vi "Hardware - ECS - EPTx Host.vi"() -> ()   [LabVIEW 2015, in "ECS-Host.lvlib"]
uses:
  ECS-Host.lvlib
  Typedefs/EPT/Engine Status.ctl
  Typedefs/EPT/Digital Channel Assignment - ECS.ctl
  ECS-Shared.lvlib
panel:
  in  "SimKnockResult":u8
  in  "PrimaryIndex":u8
  in  "Aux1Index":u8
  in  "Aux2Index":u8
  in  "Aux3Index":u8
  in  "Aux4Index":u8
  in  "PrimaryIndex2":u8
  in  "Aux1Index2":u8
  in  "Aux2Index2":u8
  in  "Aux3Index2":u8
  in  "Aux4Index2":u8
  out "EngineStatus":u8
  out "KnockResult":u8
  in  "GateReset":u8
  in  "EncoderB":u8
  in  "EncoderZ":u8
  in  "EncoderA":u8
  in  "_EPT Tab Control":T1(tab)
  in  "ForceSafeState":bool
  in  "MaxSampleRate":sgl caption="[Hz]" format="%#.3p"
  in  "EncToothCount":u32 caption="[ppr]"
  out "CurrentCAD":sgl caption="CAD" max=200 step=1
  out "ConfigFPGA2":bool caption="FPGA2Write"
  out "ConfigFPGA1":bool caption="FPGA1Write"
  in  "Aux4Filt":sgl caption="[s]" format="%#.3f"
  in  "Aux3Filt":sgl caption="[s]" format="%#.3f"
  in  "Aux2Filt":sgl caption="[s]" format="%#.3f"
  in  "Aux1Filt":sgl caption="[s]" format="%#.3f"
  in  "PrimaryFilt":sgl caption="[s]" format="%#.3f"
  out "ReceivingPrimaryFPGA2":bool caption="RCVG PRIMARY"
  out "ReceivingPrimaryFPGA1":bool caption="RCVG PRIMARY"
  out "StalledFPGA2":bool
  out "StalledFPGA1":bool
  out "AuxWarningFPGA2":bool
  out "EPTxErrorFPGA2":bool
  out "AuxWarningFPGA1":bool
  in  "SimEnable":bool
  in  "_GateReset":T2 caption="GateReset" items=["Not Selected", "9411 Chan 0", "9411 Chan 1", "9411 Chan 2", "9411 Chan 3", "9411 Chan 4", "9411 Chan 5", "AD Combo VR 1", "AD Combo VR 2", "AD Combo Hall 1", "AD Combo Hall 2"]
  in  "_EncoderZ":T2 caption="EncoderZ" items=["Not Selected", "9411 Chan 0", "9411 Chan 1", "9411 Chan 2", "9411 Chan 3", "9411 Chan 4", "9411 Chan 5", "AD Combo VR 1", "AD Combo VR 2", "AD Combo Hall 1", "AD Combo Hall 2"]
  in  "_EncoderB":T2 caption="EncoderB" items=["Not Selected", "9411 Chan 0", "9411 Chan 1", "9411 Chan 2", "9411 Chan 3", "9411 Chan 4", "9411 Chan 5", "AD Combo VR 1", "AD Combo VR 2", "AD Combo Hall 1", "AD Combo Hall 2"]
  out "SyncFPGA2":bool caption="FPGA2Sync"
  out "FPGA1Error":bool caption="FPGA1Interface"
  out "FPGA2Error":bool caption="FPGA2Interface"
  out "EngineSpeedFPGA2":sgl caption="RPM" min=0 max=0.2 step=0.001 format="%#.3f"
  in  "EncSignalSelect":bool caption="CASEncSignalSelect"
  out "WatchdogErrorFPGA1":bool
  out "OverflowFPGA1":bool
  out "PatternErrorFPGA1":bool
  out "RatioErrorFPGA1":bool
  in  "CrankRunThreshold":sgl caption="RPM" format="%#.3f"
  in  "StallSpeed":sgl caption="RPM" format="%#.3f"
  out "SyncFPGA1":bool caption="FPGA1Sync"
  out "EngineSpeedFPGA1":sgl caption="RPM" min=0 max=0.2 step=0.001 format="%#.3f"
  out "MaxCAD":sgl caption="CAD" max=200 step=1
  out "_Engine Status":T3 caption="Engine Status"
  in  "SimulatedSpeed":sgl caption="RPM" format="%#.3f"
  in  "ClearEPTxErrors":bool
  in  "SyncEnable":bool
  in  "_EncoderA":T2 caption="EncoderA" items=["Not Selected", "9411 Chan 0", "9411 Chan 1", "9411 Chan 2", "9411 Chan 3", "9411 Chan 4", "9411 Chan 5", "AD Combo VR 1", "AD Combo VR 2", "AD Combo Hall 1", "AD Combo Hall 2"]
  in  "SettingsFilename":string
  in  "ReloadEPTxSettings":bool
  out "LoadingFPGA1":bool caption="Status"
  in  "_Dig Select Tabs":enum32{"FPGA1", "FPGA2"}(tab)
  in  "_Aux4Index":T2 caption="Aux4Index" items=["Not Selected", "9411 Chan 0", "9411 Chan 1", "9411 Chan 2", "9411 Chan 3", "9411 Chan 4", "9411 Chan 5", "AD Combo VR 1", "AD Combo VR 2", "AD Combo Hall 1", "AD Combo Hall 2"]
  in  "_Aux3Index":T2 caption="Aux3Index" items=["Not Selected", "9411 Chan 0", "9411 Chan 1", "9411 Chan 2", "9411 Chan 3", "9411 Chan 4", "9411 Chan 5", "AD Combo VR 1", "AD Combo VR 2", "AD Combo Hall 1", "AD Combo Hall 2"]
  in  "_Aux2Index":T2 caption="Aux2Index" items=["Not Selected", "9411 Chan 0", "9411 Chan 1", "9411 Chan 2", "9411 Chan 3", "9411 Chan 4", "9411 Chan 5", "AD Combo VR 1", "AD Combo VR 2", "AD Combo Hall 1", "AD Combo Hall 2"]
  in  "_Aux1Index":T2 caption="Aux1Index" items=["Not Selected", "9411 Chan 0", "9411 Chan 1", "9411 Chan 2", "9411 Chan 3", "9411 Chan 4", "9411 Chan 5", "AD Combo VR 1", "AD Combo VR 2", "AD Combo Hall 1", "AD Combo Hall 2"]
  in  "_PrimaryIndex":T2 caption="PrimaryIndex" items=["Not Selected", "9411 Chan 0", "9411 Chan 1", "9411 Chan 2", "9411 Chan 3", "9411 Chan 4", "9411 Chan 5", "AD Combo VR 1", "AD Combo VR 2", "AD Combo Hall 1", "AD Combo Hall 2"]
  in  "_Aux4Index2":T2 caption="Aux4Index" items=["Not Selected", "9411 Chan 0", "9411 Chan 1", "9411 Chan 2", "9411 Chan 3", "9411 Chan 4", "9411 Chan 5", "AD Combo VR 1", "AD Combo VR 2", "AD Combo Hall 1", "AD Combo Hall 2"]
  in  "_Aux3Index2":T2 caption="Aux3Index" items=["Not Selected", "9411 Chan 0", "9411 Chan 1", "9411 Chan 2", "9411 Chan 3", "9411 Chan 4", "9411 Chan 5", "AD Combo VR 1", "AD Combo VR 2", "AD Combo Hall 1", "AD Combo Hall 2"]
  in  "_Aux2Index2":T2 caption="Aux2Index" items=["Not Selected", "9411 Chan 0", "9411 Chan 1", "9411 Chan 2", "9411 Chan 3", "9411 Chan 4", "9411 Chan 5", "AD Combo VR 1", "AD Combo VR 2", "AD Combo Hall 1", "AD Combo Hall 2"]
  in  "_Aux1Index2":T2 caption="Aux1Index" items=["Not Selected", "9411 Chan 0", "9411 Chan 1", "9411 Chan 2", "9411 Chan 3", "9411 Chan 4", "9411 Chan 5", "AD Combo VR 1", "AD Combo VR 2", "AD Combo Hall 1", "AD Combo Hall 2"]
  in  "_PrimaryIndex2":T2 caption="PrimaryIndex" items=["Not Selected", "9411 Chan 0", "9411 Chan 1", "9411 Chan 2", "9411 Chan 3", "9411 Chan 4", "9411 Chan 5", "AD Combo VR 1", "AD Combo VR 2", "AD Combo Hall 1", "AD Combo Hall 2"]
  in  "AuxTTL-3TDC":T4(ring)
  in  "AuxTTL-4TDC":T4(ring)
  in  "AuxTTL-7TDC":T4(ring)
  in  "AuxTTL-8TDC":T4(ring)
  in  "AuxTTL-2TDC":T4(ring)
  in  "AuxTTL-1TDC":T4(ring)
  in  "AuxTTL-5TDC":T4(ring)
  in  "AuxTTL-6TDC":T4(ring)
  in  "Spark1-3TDC":T4(ring)
  in  "Spark1-4TDC":T4(ring)
  in  "Spark1-7TDC":T4(ring)
  in  "Spark1-8TDC":T4(ring)
  in  "Spark1-2TDC":T4(ring)
  in  "Spark1-1TDC":T4(ring)
  in  "Spark1-5TDC":T4(ring)
  in  "Spark1-6TDC":T4(ring)
  in  "DI1-2TDC":T4(ring)
  in  "DI1-1TDC":T4(ring)
  in  "DI2-2TDC":T4(ring)
  in  "DI2-1TDC":T4(ring)
  in  "DI4-2TDC":T4(ring)
  in  "DI4-1TDC":T4(ring)
  in  "DI3-2TDC":T4(ring)
  in  "DI3-1TDC":T4(ring)
  in  "GlobalTDCOffset":sgl caption="CAD" min=0 max=0.2 step=0.001 format="%#.3f"
  in  "TDC1":sgl caption="CAD" min=0 max=720 step=0.001 format="%#.3f"
  in  "TDC2":sgl caption="CAD" min=0 max=720 step=0.001 format="%#.3f"
  in  "TDC3":sgl caption="CAD" min=0 max=720 step=0.001 format="%#.3f"
  in  "TDC4":sgl caption="CAD" min=0 max=0.2 step=0.001 format="%#.3f"
  in  "TDC5":sgl caption="CAD" min=0 max=0.2 step=0.001 format="%#.3f"
  in  "TDC6":sgl caption="CAD" min=0 max=0.2 step=0.001 format="%#.3f"
  in  "TDC7":sgl caption="CAD" min=0 max=0.2 step=0.001 format="%#.3f"
  in  "TDC8":sgl caption="CAD" min=0 max=0.2 step=0.001 format="%#.3f"
  in  "PFI1-3TDC":T4(ring)
  in  "PFI1-4TDC":T4(ring)
  in  "PFI2-3TDC":T4(ring)
  in  "PFI2-4TDC":T4(ring)
  in  "PFI1-2TDC":T4(ring)
  in  "PFI1-1TDC":T4(ring)
  in  "PFI2-1TDC":T4(ring)
  in  "PFI2-2TDC":T4(ring)
  out "Aux4EdgeCount":sgl caption="[DBTDC]"
  out "Aux3EdgeCount":sgl caption="[]"
  out "Aux2EdgeCount":sgl caption="[]"
  out "Aux1EdgeCount":sgl caption="[]"
  out "Aux4Adv":sgl caption="[CAD]" format="%#.2f"
  in  "Aux4DefaultPsn":sgl caption="[DBTDC]" format="%#.2f"
  out "Aux4RisingEdge":sgl caption="[DBTDC]"
  in  "Aux4CaptureStart":sgl caption="[DBTDC]" format="%#.2f"
  in  "Aux4CaptureEnd":sgl caption="[DBTDC]" format="%#.2f"
  out "Aux3Adv":sgl caption="[CAD]" format="%#.2f"
  in  "Aux3DefaultPsn":sgl caption="[DBTDC]" format="%#.2f"
  out "Aux3RisingEdge":sgl caption="[]"
  in  "Aux3CaptureStart":sgl caption="[DBTDC]" format="%#.2f"
  in  "Aux3CaptureEnd":sgl caption="[]" format="%#.2f"
  out "Aux2Adv":sgl caption="[CAD]" format="%#.2f"
  out "Aux1Adv":sgl caption="[CAD]" format="%#.2f"
  in  "Aux2DefaultPsn":sgl caption="[DBTDC]" format="%#.2f"
  in  "Aux1DefaultPsn":sgl caption="[DBTDC]" format="%#.2f"
  out "Aux2RisingEdge":sgl caption="[]"
  out "Aux1RisingEdge":sgl caption="[]"
  in  "Aux1CaptureStart":sgl caption="[DBTDC]" format="%#.2f"
  in  "Aux1CaptureEnd":sgl caption="[]" format="%#.2f"
  in  "Aux2CaptureStart":sgl caption="[DBTDC]" format="%#.2f"
  in  "Aux2CaptureEnd":sgl caption="[]" format="%#.2f"
  in  "VVT-TDCRef":T5(ring)
  in  "SimKnockEnable":bool
  in  "_SimKnockResult":bool[](array[boolean]) caption="SimKnockResult"
  in  "Knock-6TDC":T4(ring)
  in  "Knock-8TDC":T4(ring)
  in  "Knock-4TDC":T4(ring)
  in  "Knock-2TDC":T4(ring)
  in  "Knock-1TDC":T4(ring)
  in  "Knock-5TDC":T4(ring)
  in  "Knock-3TDC":T4(ring)
  in  "Knock-7TDC":T4(ring)
  in  "KnockSensorCyl3":T4(ring)
  in  "KnockSensorCyl4":T4(ring)
  in  "KnockSensorCyl7":T4(ring)
  in  "KnockSensorCyl8":T4(ring)
  in  "KnockSensorCyl2":T4(ring)
  in  "KnockSensorCyl1":T4(ring)
  in  "KnockSensorCyl5":T4(ring)
  in  "KnockSensorCyl6":T4(ring)
  in  "KnockRefWindowEnd":sgl caption="[DBTDC]"
  in  "KnockRefWindowStart":sgl caption="[DBTDC]"
  in  "KnockWindowEnd":sgl caption="[DBTDC]"
  in  "KnockWindowStart":sgl caption="[DBTDC]"
  in  "KnockThreshold":sgl caption="[]"
  in  "KnockHighCutoff":sgl caption="[Hz]"
  in  "KnockLowCutoff":sgl caption="[Hz]"
  in  "KnockFrequency":sgl caption="[Hz]"
  out "KnockIntensity":sgl[](array[numeric])
  out "_Knock":bool[](array[boolean]) caption="Knock"
  # "FPGA1"
  # "FPGA2"
  # "FPGA1"
  # "FPGA2"
  # "Sim Encoder\nResolution"
  # "Max CAS DAQ\nSample Rate"
  # "Digital Signal and Filter Select"
  # "AUX 1"
  # "AUX 2"
  # "AUX 3"
  # "AUX 4"
  # "CaptureStart"
  # "CaptureEnd"
  # "RisingEdge"
  # "EdgeCount"
  # "DefaultPosition"
  # "Advance"
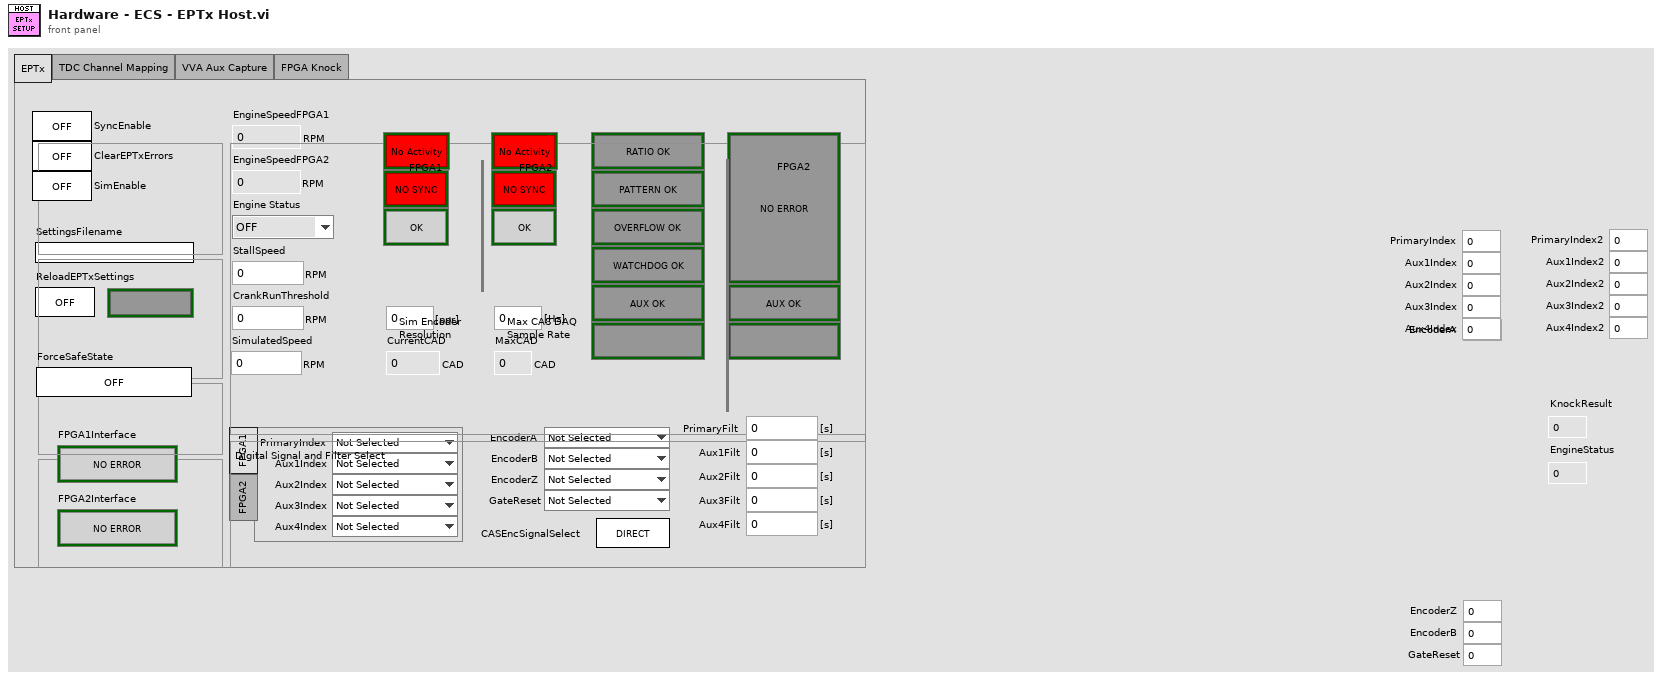
[diagram p1: front panel]
types:
  T1 = enum32{"EPTx", "TDC Channel Mapping", "VVA Aux Capture", "FPGA Knock"}
  T2 = typedef "ECS-Shared.lvlib/Digital Channel Assignment - ECS.ctl" = u8
  T3 = typedef "ECS-Shared.lvlib/Engine Status.ctl" = enum16{"OFF", "STALLED", "CRANKING", "RUNNING", "ACCEL", "DECEL", "SAFE"}
  T4 = enum32{"TDC1", "TDC2", "TDC3", "TDC4", "TDC5", "TDC6", "TDC7", "TDC8", "TDC9", "TDC10", "TDC11", "TDC12"}
  T5 = enum32{"TDC1", "TDC2", "TDC3", "TDC4", "TDC5", "TDC6", "TDC7", "TDC8"}
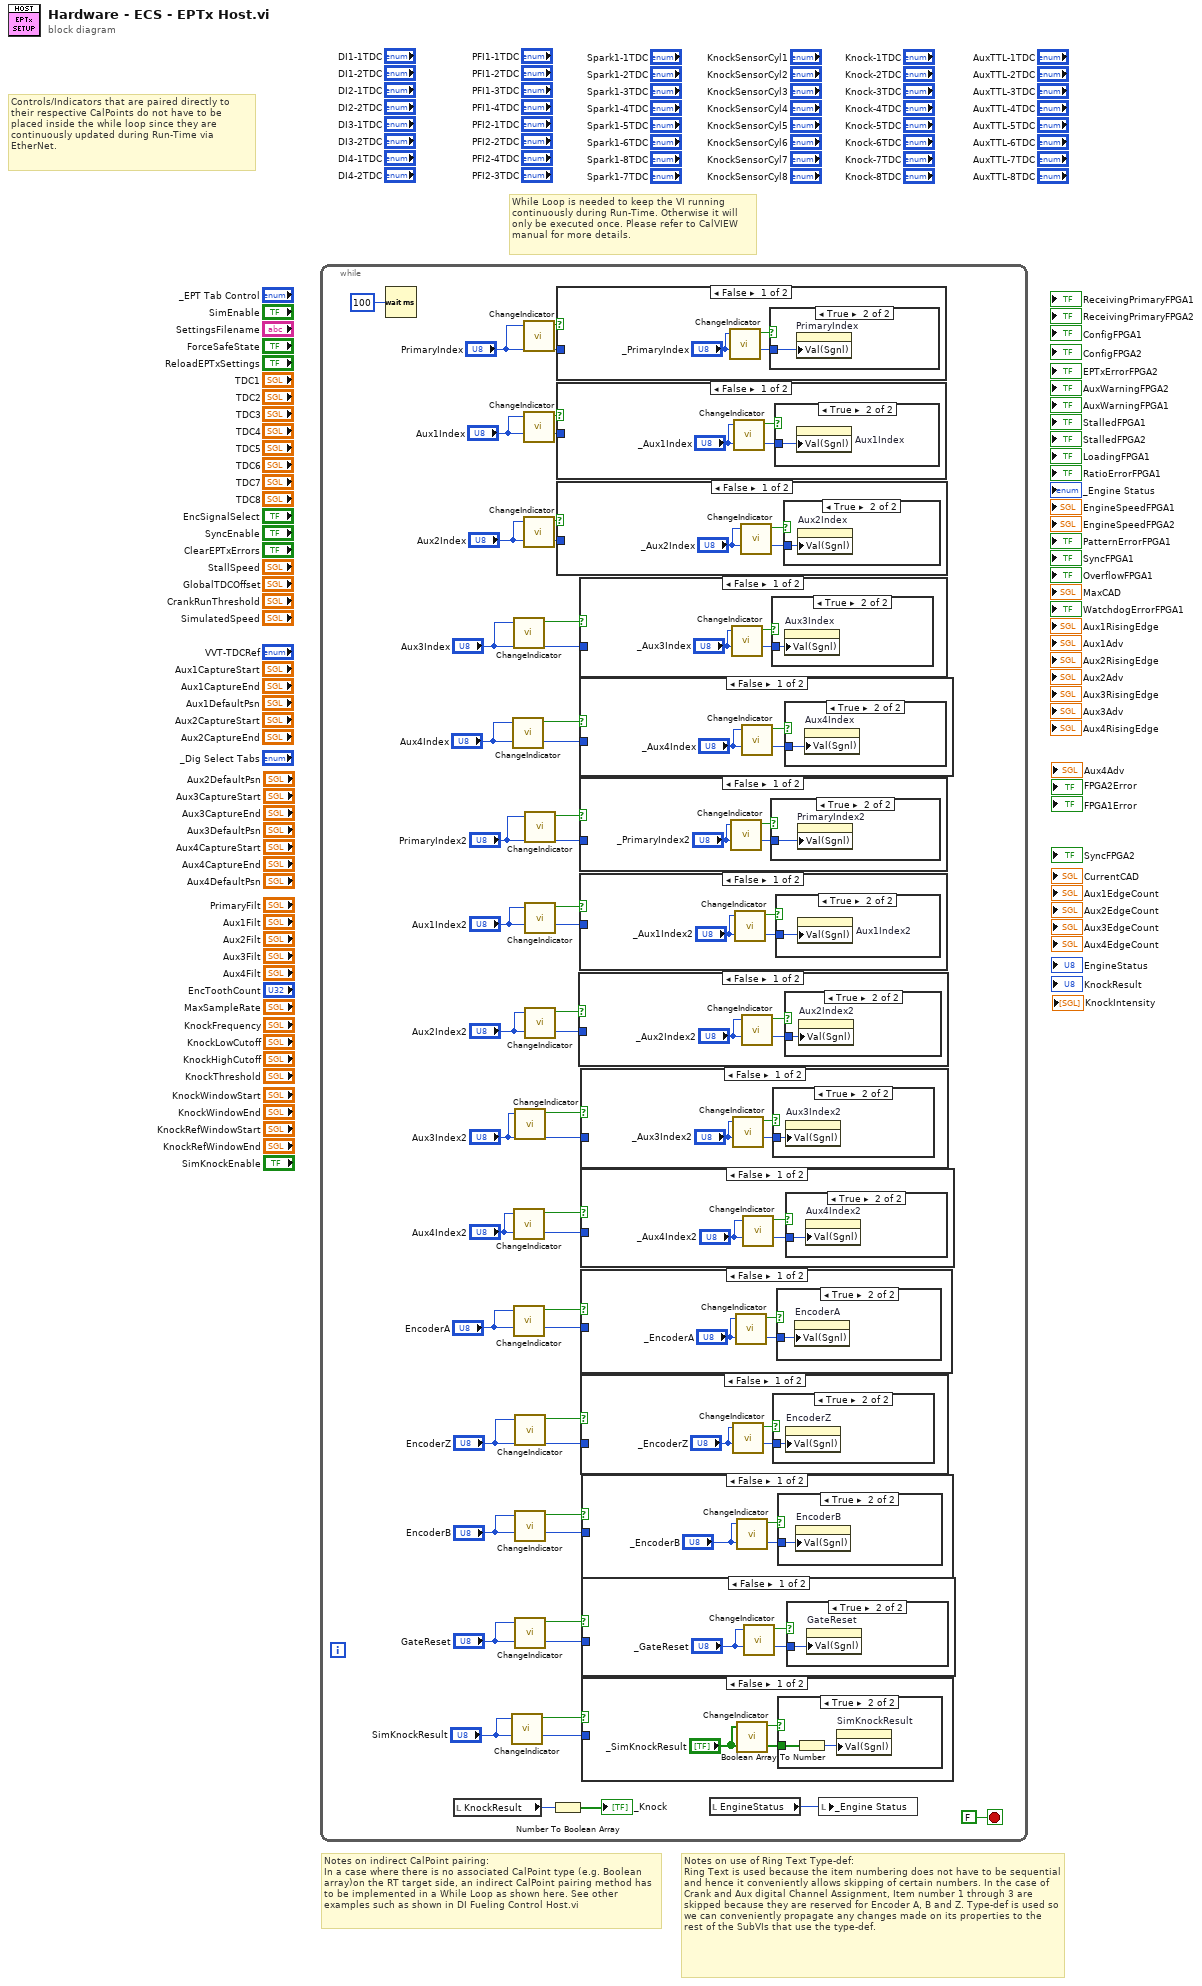
[diagram p0: block diagram]
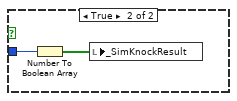
[diagram p3: hidden frame]
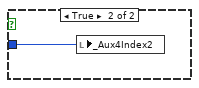
[diagram p5: hidden frame]
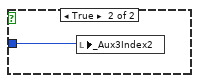
[diagram p7: hidden frame]
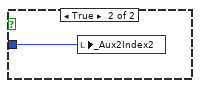
[diagram p9: hidden frame]
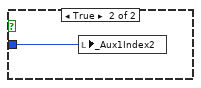
[diagram p11: hidden frame]
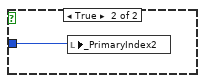
[diagram p13: hidden frame]
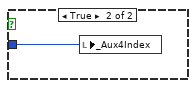
[diagram p15: hidden frame]
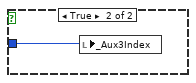
[diagram p17: hidden frame]
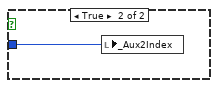
[diagram p19: hidden frame]
diagram:
  # "Controls/Indicators that are paired directly to their respective CalPoints do not have to be placed inside the while loop since they are continuously updated during Run-Time via EtherNet."
  # "While Loop is needed to keep the VI running\ncontinuously during Run-Time. Otherwise it will only be executed once. Please refer to CalVIEW manual for more details."
  # "Notes on use of Ring Text Type-def:\nRing Text is used because the item numbering does not have to be sequential and hence it conveniently allows skipping of certain numbers. In the case of Crank and Aux digital Channel Assignment, Item number 1 through 3 are skipped because they are reserved for Encoder A, B and Z. Type-def is used so we can conveniently propagate any changes made on its properties to the rest of the SubVIs that use the type-def."
  # "Notes on indirect CalPoint pairing:\nIn a case where there is no associated CalPoint type (e.g. Boolean array)on the RT target side, an indirect CalPoint pairing method has to be implemented in a While Loop as shown here. See other examples such as shown in DI Fueling Control Host.vi"
  n1 = while {
    stop <- FALSE stop-if-true
    n2 = Wait (ms)(milliseconds to wait=u32 100 ("millisecond timer value")) -> ()  [unwired: 1 out]
    n3 = local read "KnockResult"() -> (w24:u8)
    n4 = call "ChangeIndicator.vi"("Input"="SimKnockResult") -> ("Change"=w1:bool)  [unwired: 9 in]
    n5 = call "ChangeIndicator.vi"("Input"="Aux4Index") -> ("Change"=w14:bool)  [unwired: 9 in]
    n6 = call "ChangeIndicator.vi"("Input"="Aux3Index") -> ("Change"=w16:bool)  [unwired: 9 in]
    n7 = call "ChangeIndicator.vi"("Input"="Aux4Index2") -> ("Change"=w11:bool)  [unwired: 9 in]
    n8 = call "ChangeIndicator.vi"("Input"="EncoderA") -> ("Change"=w33:bool)  [unwired: 9 in]
    n9 = call "ChangeIndicator.vi"("Input"="Aux3Index2") -> ("Change"=w9:bool)  [unwired: 9 in]
    n10 = call "ChangeIndicator.vi"("Input"="EncoderZ") -> ("Change"=w26:bool)  [unwired: 9 in]
    n11 = call "ChangeIndicator.vi"("Input"="EncoderB") -> ("Change"=w27:bool)  [unwired: 9 in]
    n12 = call "ChangeIndicator.vi"("Input"="GateReset") -> ("Change"=w28:bool)  [unwired: 9 in]
    n13 = call "ChangeIndicator.vi"("Input"="PrimaryIndex") -> ("Change"=w21:bool)  [unwired: 9 in]
    n14 = call "ChangeIndicator.vi"("Input"="Aux1Index") -> ("Change"=w20:bool)  [unwired: 9 in]
    n15 = call "ChangeIndicator.vi"("Input"="Aux2Index") -> ("Change"=w18:bool)  [unwired: 9 in]
    n16 = call "ChangeIndicator.vi"("Input"="PrimaryIndex2") -> ("Change"=w4:bool)  [unwired: 9 in]
    n17 = call "ChangeIndicator.vi"("Input"="Aux1Index2") -> ("Change"=w5:bool)  [unwired: 9 in]
    n18 = call "ChangeIndicator.vi"("Input"="Aux2Index2") -> ("Change"=w7:bool)  [unwired: 9 in]
    n19 = Number To Boolean Array(number=w24) -> (Boolean array=→"_Knock":bool[])
    n20 = case shown="False" w21 {
      tunnel: "PrimaryIndex" -> [_ w81]
      frame False {
        n21 = call "ChangeIndicator.vi"("Input"="_PrimaryIndex") -> ("Change"=w79:bool)  [unwired: 9 in]
        n22 = case shown="True" w79 {
          tunnel: "_PrimaryIndex" -> [_ w80]
          frame False {
          }
          frame True {
            n23 = property on="PrimaryIndex" class="DigNum (strict)"("Val(Sgnl)"=w80) -> ()  [unwired: 2 in, 2 out]
          }
        }
      }
      frame True {
        n24 = local write "_PrimaryIndex"(w81) -> ()
      }
    }
    n25 = case shown="False" w20 {
      tunnel: "Aux1Index" -> [_ w77]
      frame False {
        n26 = call "ChangeIndicator.vi"("Input"="_Aux1Index") -> ("Change"=w75:bool)  [unwired: 9 in]
        n27 = case shown="True" w75 {
          tunnel: "_Aux1Index" -> [_ w76]
          frame False {
          }
          frame True {
            n28 = property on="Aux1Index" class="DigNum (strict)"("Val(Sgnl)"=w76) -> ()  [unwired: 2 in, 2 out]
          }
        }
      }
      frame True {
        n29 = local write "_Aux1Index"(w77) -> ()
      }
    }
    n30 = case shown="False" w18 {
      tunnel: "Aux2Index" -> [_ w73]
      frame False {
        n31 = call "ChangeIndicator.vi"("Input"="_Aux2Index") -> ("Change"=w71:bool)  [unwired: 9 in]
        n32 = case shown="True" w71 {
          tunnel: "_Aux2Index" -> [_ w72]
          frame False {
          }
          frame True {
            n33 = property on="Aux2Index" class="DigNum (strict)"("Val(Sgnl)"=w72) -> ()  [unwired: 2 in, 2 out]
          }
        }
      }
      frame True {
        n34 = local write "_Aux2Index"(w73) -> ()
      }
    }
    n35 = case shown="False" w7 {
      tunnel: "Aux2Index2" -> [_ w53]
      frame False {
        n36 = call "ChangeIndicator.vi"("Input"="_Aux2Index2") -> ("Change"=w51:bool)  [unwired: 9 in]
        n37 = case shown="True" w51 {
          tunnel: "_Aux2Index2" -> [_ w52]
          frame False {
          }
          frame True {
            n38 = property on="Aux2Index2" class="DigNum (strict)"("Val(Sgnl)"=w52) -> ()  [unwired: 2 in, 2 out]
          }
        }
      }
      frame True {
        n39 = local write "_Aux2Index2"(w53) -> ()
      }
    }
    n40 = case shown="False" w16 {
      tunnel: "Aux3Index" -> [_ w69]
      frame False {
        n41 = call "ChangeIndicator.vi"("Input"="_Aux3Index") -> ("Change"=w67:bool)  [unwired: 9 in]
        n42 = case shown="True" w67 {
          tunnel: "_Aux3Index" -> [_ w68]
          frame False {
          }
          frame True {
            n43 = property on="Aux3Index" class="DigNum (strict)"("Val(Sgnl)"=w68) -> ()  [unwired: 2 in, 2 out]
          }
        }
      }
      frame True {
        n44 = local write "_Aux3Index"(w69) -> ()
      }
    }
    n45 = case shown="False" w14 {
      tunnel: "Aux4Index" -> [_ w65]
      frame False {
        n46 = call "ChangeIndicator.vi"("Input"="_Aux4Index") -> ("Change"=w63:bool)  [unwired: 9 in]
        n47 = case shown="True" w63 {
          tunnel: "_Aux4Index" -> [_ w64]
          frame False {
          }
          frame True {
            n48 = property on="Aux4Index" class="DigNum (strict)"("Val(Sgnl)"=w64) -> ()  [unwired: 2 in, 2 out]
          }
        }
      }
      frame True {
        n49 = local write "_Aux4Index"(w65) -> ()
      }
    }
    n50 = case shown="False" w4 {
      tunnel: "PrimaryIndex2" -> [_ w61]
      frame False {
        n51 = call "ChangeIndicator.vi"("Input"="_PrimaryIndex2") -> ("Change"=w59:bool)  [unwired: 9 in]
        n52 = case shown="True" w59 {
          tunnel: "_PrimaryIndex2" -> [_ w60]
          frame False {
          }
          frame True {
            n53 = property on="PrimaryIndex2" class="DigNum (strict)"("Val(Sgnl)"=w60) -> ()  [unwired: 2 in, 2 out]
          }
        }
      }
      frame True {
        n54 = local write "_PrimaryIndex2"(w61) -> ()
      }
    }
    n55 = case shown="False" w5 {
      tunnel: "Aux1Index2" -> [_ w57]
      frame False {
        n56 = call "ChangeIndicator.vi"("Input"="_Aux1Index2") -> ("Change"=w55:bool)  [unwired: 9 in]
        n57 = case shown="True" w55 {
          tunnel: "_Aux1Index2" -> [_ w56]
          frame False {
          }
          frame True {
            n58 = property on="Aux1Index2" class="DigNum (strict)"("Val(Sgnl)"=w56) -> ()  [unwired: 2 in, 2 out]
          }
        }
      }
      frame True {
        n59 = local write "_Aux1Index2"(w57) -> ()
      }
    }
    n60 = case shown="False" w9 {
      tunnel: "Aux3Index2" -> [_ w49]
      frame False {
        n61 = call "ChangeIndicator.vi"("Input"="_Aux3Index2") -> ("Change"=w47:bool)  [unwired: 9 in]
        n62 = case shown="True" w47 {
          tunnel: "_Aux3Index2" -> [_ w48]
          frame False {
          }
          frame True {
            n63 = property on="Aux3Index2" class="DigNum (strict)"("Val(Sgnl)"=w48) -> ()  [unwired: 2 in, 2 out]
          }
        }
      }
      frame True {
        n64 = local write "_Aux3Index2"(w49) -> ()
      }
    }
    n65 = case shown="False" w11 {
      tunnel: "Aux4Index2" -> [_ w45]
      frame False {
        n66 = call "ChangeIndicator.vi"("Input"="_Aux4Index2") -> ("Change"=w43:bool)  [unwired: 9 in]
        n67 = case shown="True" w43 {
          tunnel: "_Aux4Index2" -> [_ w44]
          frame False {
          }
          frame True {
            n68 = property on="Aux4Index2" class="DigNum (strict)"("Val(Sgnl)"=w44) -> ()  [unwired: 2 in, 2 out]
          }
        }
      }
      frame True {
        n69 = local write "_Aux4Index2"(w45) -> ()
      }
    }
    n70 = case shown="False" w33 {
      tunnel: "EncoderA" -> [_ w97]
      frame False {
        n71 = call "ChangeIndicator.vi"("Input"="_EncoderA") -> ("Change"=w95:bool)  [unwired: 9 in]
        n72 = case shown="True" w95 {
          tunnel: "_EncoderA" -> [_ w96]
          frame False {
          }
          frame True {
            n73 = property on="EncoderA" class="DigNum (strict)"("Val(Sgnl)"=w96) -> ()  [unwired: 2 in, 2 out]
          }
        }
      }
      frame True {
        n74 = local write "_EncoderA"(w97) -> ()
      }
    }
    n75 = case shown="False" w26 {
      tunnel: "EncoderZ" -> [_ w93]
      frame False {
        n76 = call "ChangeIndicator.vi"("Input"="_EncoderZ") -> ("Change"=w91:bool)  [unwired: 9 in]
        n77 = case shown="True" w91 {
          tunnel: "_EncoderZ" -> [_ w92]
          frame False {
          }
          frame True {
            n78 = property on="EncoderZ" class="DigNum (strict)"("Val(Sgnl)"=w92) -> ()  [unwired: 2 in, 2 out]
          }
        }
      }
      frame True {
        n79 = local write "_EncoderZ"(w93) -> ()
      }
    }
    n80 = case shown="False" w27 {
      tunnel: "EncoderB" -> [_ w89]
      frame False {
        n81 = call "ChangeIndicator.vi"("Input"="_EncoderB") -> ("Change"=w87:bool)  [unwired: 9 in]
        n82 = case shown="True" w87 {
          tunnel: "_EncoderB" -> [_ w88]
          frame False {
          }
          frame True {
            n83 = property on="EncoderB" class="DigNum (strict)"("Val(Sgnl)"=w88) -> ()  [unwired: 2 in, 2 out]
          }
        }
      }
      frame True {
        n84 = local write "_EncoderB"(w89) -> ()
      }
    }
    n85 = case shown="False" w28 {
      tunnel: "GateReset" -> [_ w85]
      frame False {
        n86 = call "ChangeIndicator.vi"("Input"="_GateReset") -> ("Change"=w83:bool)  [unwired: 9 in]
        n87 = case shown="True" w83 {
          tunnel: "_GateReset" -> [_ w84]
          frame False {
          }
          frame True {
            n88 = property on="GateReset" class="DigNum (strict)"("Val(Sgnl)"=w84) -> ()  [unwired: 2 in, 2 out]
          }
        }
      }
      frame True {
        n89 = local write "_GateReset"(w85) -> ()
      }
    }
    n90 = case shown="False" w1 {
      tunnel: "SimKnockResult" -> [_ w41]
      frame False {
        n91 = call "ChangeIndicator.vi"("Input"="_SimKnockResult") -> ("Change"=w37:bool)  [unwired: 9 in]
        n92 = case shown="True" w37 {
          tunnel: "_SimKnockResult" -> [_ w39]
          frame False {
          }
          frame True {
            n93 = Boolean Array To Number(Boolean array=w39) -> (number=w38:u32)
            n94 = property on="SimKnockResult" class="DigNum (strict)"("Val(Sgnl)"=w38) -> ()  [unwired: 2 in, 2 out]
          }
        }
      }
      frame True {
        n95 = Number To Boolean Array(number=w41) -> (Boolean array=w40:bool[])
        n96 = local write "_SimKnockResult"(w40) -> ()
      }
    }
    n97 = local read "EngineStatus"() -> (w25:u8)
    n98 = local write "_Engine Status"(w25) -> ()
  }
